vi "Read Direction.vi"(8 "error in (no error)":errorcluster, 11 "Mouse in":refnum<class "Mouse.lvclass">) -> (0 "error out":errorcluster, 2 "Direction":T1, 3 "Mouse out":refnum<class "Mouse.lvclass">)   [LabVIEW 2021, in "Mouse.lvclass"]
uses:
  Mouse.lvclass
  GameEl_class/private/Enum Direction.ctl
  Mouse.lvclass/Mouse.ctl
  GameEl_class/GameEl.lvclass
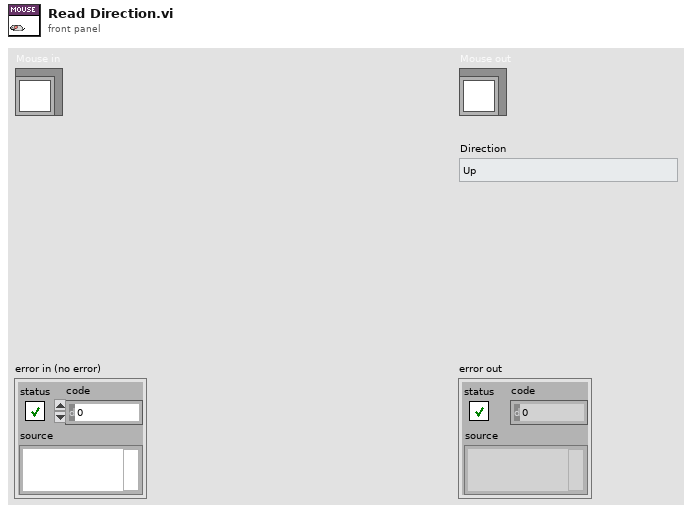
[diagram p1: front panel]
types:
  T1 = typedef "GameEl.lvclass/Enum Direction.ctl" = enum16{"Up", "Down", "Forward", "Backward"}
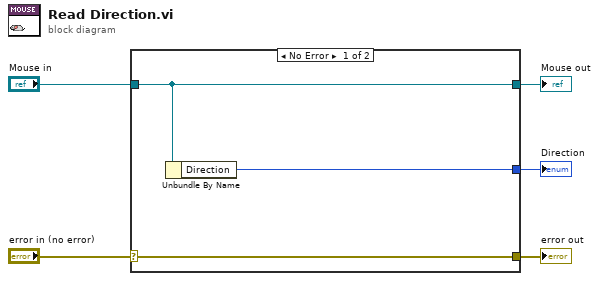
[diagram p0: block diagram]
diagram:
  n1 = case shown="No Error" "error in (no error)" {
    selector: "error in (no error)" -> [w8 w9]
    tunnel: [w8 w9] -> w4
    tunnel: [w7 w10] -> w2
    tunnel: "Mouse in" -> [w7 w10]
    tunnel: [w6 _] -> w1
    frame No Error {
      n2 = Unbundle By Name(w7) -> ("Direction"=w6:T1)
    }
    frame Error {
    }
  }
  "error out" <- w4
  "Mouse out" <- w2
  "Direction" <- w1
